vi "Get IPs and subnet masks.vi"(8 "error in (no error)":errorcluster) -> (0 "error out":errorcluster, 1 "standard output":string, 2 "Array 2":string[](array[string]), 3 "Array":string[](array[string]))   [LabVIEW 2020]
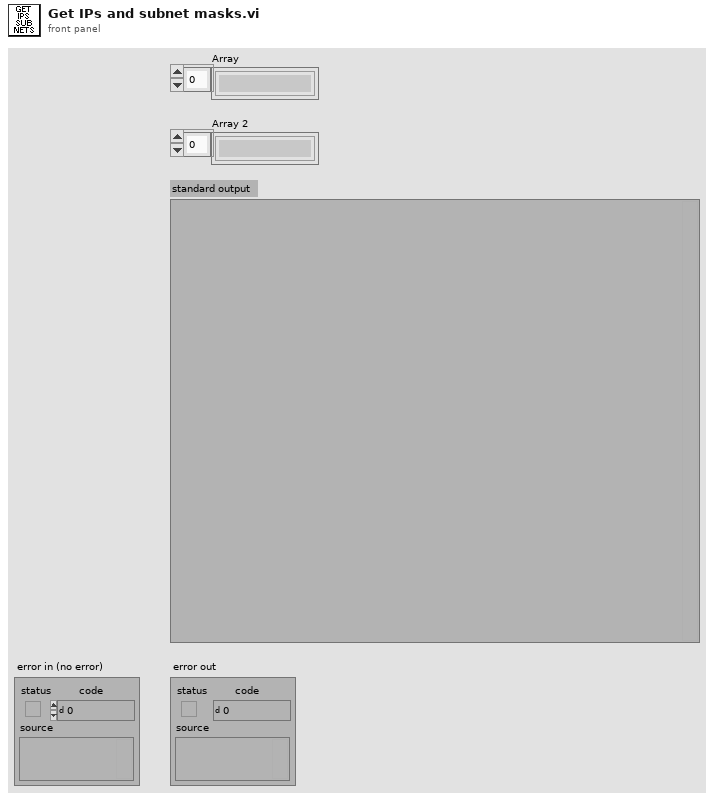
[diagram p1: front panel]
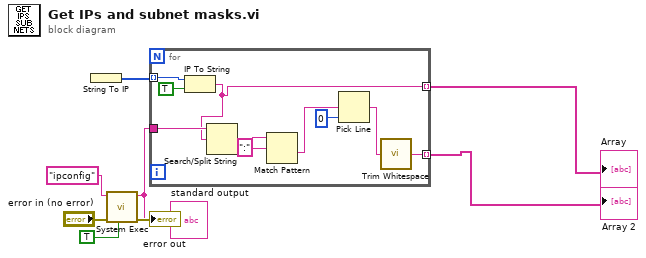
[diagram p0: block diagram]
diagram:
  n1 = String To IP() -> (0:w6:u32[])  [unwired: 1 in]
  n2 = call "System Exec.vi"("run minimized? (F)"=TRUE, "error in (no error)"="error in (no error)", "command line"="ipconfig") -> ("error out"=→"error out":errorcluster, "standard output"=w3:string)  [unwired: 5 in, 2 out]
  "standard output" <- w3
  n3 = for {
    tunnel: [w17] -> w7 mode=indexing
    tunnel: w3 -> [w16]
    tunnel: w6 -> [w10] mode=indexing
    tunnel: [w9] -> w8 mode=indexing
    n4 = IP To String(1:TRUE ("dot notation? (F)"), 2:w10) -> (0:w9:string)
    n5 = Search/Split String(string=w16, search string/char (-)=w9) -> (match + rest of string=w15:string)  [unwired: 1 in, 2 out]
    n6 = Match Pattern(string=w15, regular expression=":") -> (after substring=w13:string)  [unwired: 1 in, 3 out]
    n7 = Pick Line(multi-line string=w13, line index=0) -> (output string=w12:string)  [unwired: 1 in]
    n8 = call "Trim Whitespace.vi"("string"=w12) -> ("trimmed string"=w17:string)  [unwired: 1 in]
  }
  "Array" <- w8
  "Array 2" <- w7
